vi "Compile Directional Speed 1.0 Data - Multi FPGA.vi"(7 "RIO Address":string, 8 "error in (no error)":errorcluster, 11 "Device Item Ref in":T3 format="%.0x") -> (0 "error out":errorcluster, 1 "bitfile names":string[](array[string]), 2 "Directional Speeds":T1[](array[typedef]), 3 "Device Item Ref out":T3 format="%.0x")   [LabVIEW 2015, in "Engine Simulation Toolkit System Explorer.lvlib"]
uses:
  Engine Simulation Toolkit System Explorer.lvlib
  <vilib>/NI Veristand/Custom Device API/Custom Device Item Ref.ctl
  Shared/1.0 Directional Speed Engine Data.ctl
  Shared/1.0 Directional Speed FIFO Idxs.ctl
  Digital Pattern Find Events Enum.ctl
  Custom wrapped 10 bit counter.vi
  Shared/Constants and GUIDs.vi
  <vilib>/NI Veristand/Custom Device Tools/Custom Device Utility Library/NI VeriStand - Search for Item by GUID.vi
  Shared/Properties.vi
  <vilib>/NI Veristand/Custom Device API/Get Item Property (String).vi
  <vilib>/NI Veristand/Custom Device API/Get Item Property (Dependent Node Pointer).vi
  <vilib>/NI Veristand/Custom Device Tools/Custom Device Utility Library/Custom Device Utility Library.lvlib
  Shared/Engine Simulation Toolkit Shared.lvlib
  <vilib>/NI Veristand/Custom Device API/Custom Device API.lvlib
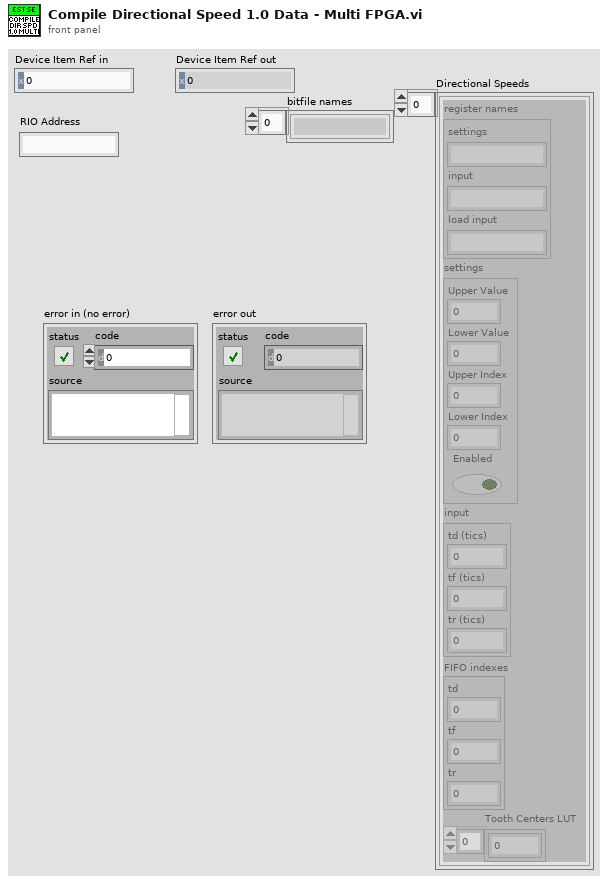
[diagram p1: front panel]
types:
  T1 = typedef "Engine Simulation Toolkit Shared.lvlib/1.0 Directional Speed Engine Data.ctl" = cluster{"register names":cluster{"settings":string, "input":string, "load input":string}, "settings":cluster{"Upper Value":u16, "Lower Value":u16, "Upper Index":fxp<+,10,10>, "Lower Index":fxp<+,10,10>, "Enabled":bool}, "input":cluster{"td (tics)":u16, "tf (tics)":u16, "tr (tics)":u16}, "FIFO indexes":T2, "Tooth Centers LUT":u16[]}
  T2 = typedef "Engine Simulation Toolkit Shared.lvlib/1.0 Directional Speed FIFO Idxs.ctl" = cluster{"td":i32, "tf":i32, "tr":i32}
  T3 = typedef "Custom Device API.lvlib/Custom Device Item Ref.ctl" = u64
  T4 = typedef "Engine Simulation Toolkit Shared.lvlib/Channel.ctl" = cluster{"Name":string, "Units":string, "Default":dbl, "Description":string, "Scalable":bool}
  T5 = typedef "Engine Simulation Toolkit System Explorer.lvlib/Digital Pattern Find Events Enum.ctl" = enum16{"Rising Edge", "Falling Edge", "Any Edge", "Center Tooth", "Center Gap"}
  T6 = typedef "Custom Device API.lvlib/Custom Device Item Info.ctl" = cluster{"Name":string, "Is Channel":bool, "GUID":string, "Is Waveform":bool}
  T7 = typedef "Engine Simulation Toolkit System Explorer.lvlib/Digital Pattern.ctl" = cluster{"Name":string, "Base":T8, "Remove":T9[], "Add":T10[], "FPGA Resource":string}
  T8 = typedef "Engine Simulation Toolkit System Explorer.lvlib/Digital Pattern Base.ctl" = cluster{"Length":dbl, "Teeth":u16, "Width":dbl, "Offset":dbl}
  T9 = typedef "Engine Simulation Toolkit System Explorer.lvlib/Digital Pattern Remove Edge.ctl" = cluster{"Tooth":u16, "Edge":bool}
  T10 = typedef "Engine Simulation Toolkit System Explorer.lvlib/Digital Pattern Add Pulse.ctl" = cluster{"Tooth":u16, "Offset":dbl, "Width":dbl}
  T11 = typedef "Engine Simulation Toolkit System Explorer.lvlib/Digital Pattern Expanded.ctl" = cluster{"X":dbl[], "Y":dbl[]}
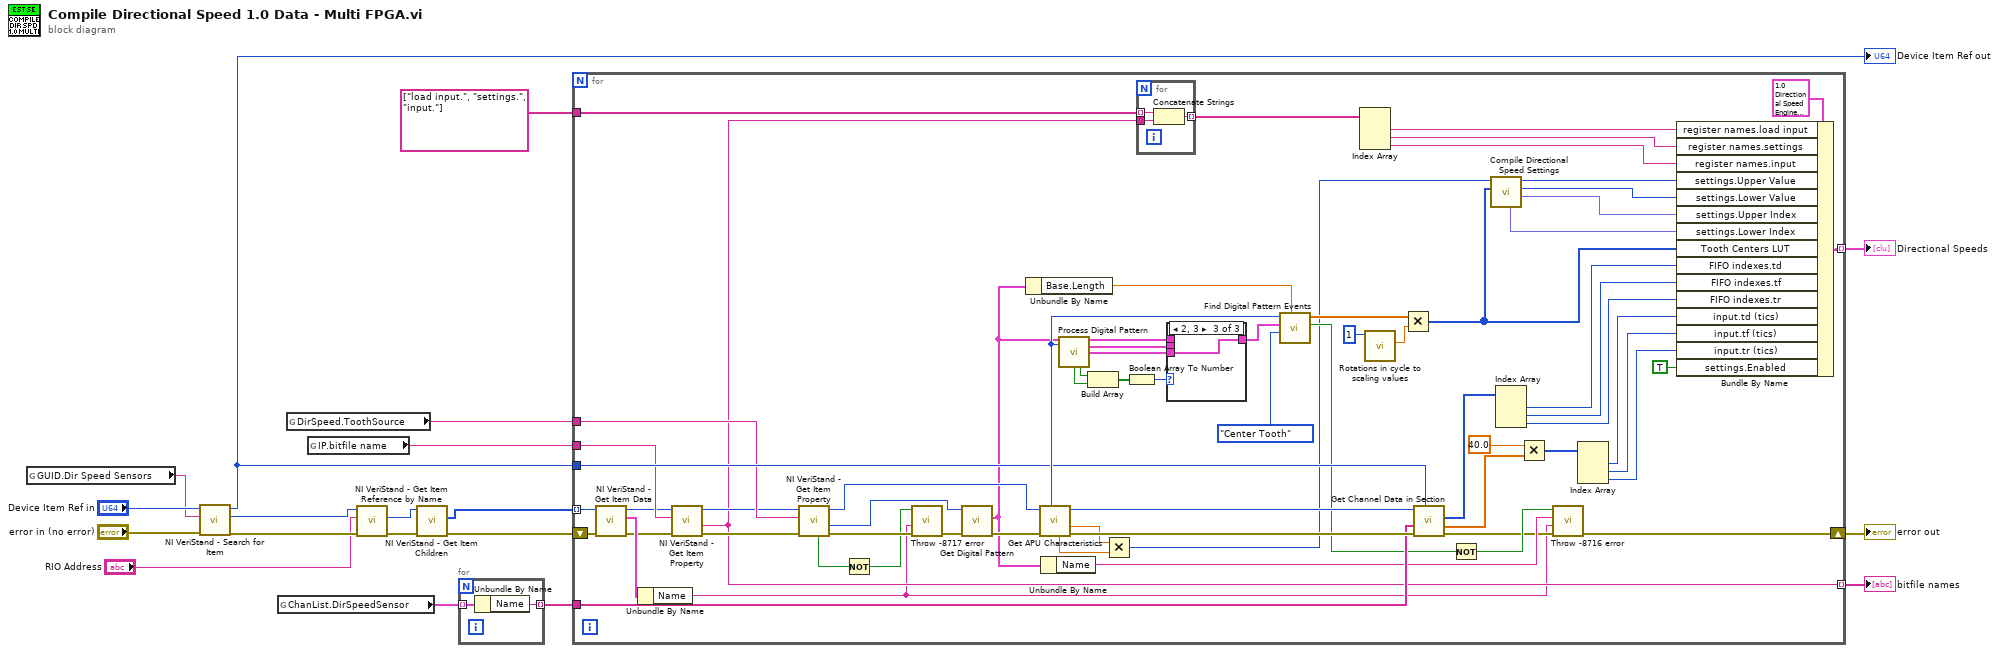
[diagram p0: block diagram]
diagram:
  n1 = global read "Constants and GUIDs.vi" "GUID.Dir Speed Sensors"() -> (w17:string)
  n2 = call-poly <vilib>:"NI VeriStand - Search for Item.vi"("error in"="error in (no error)", "Item GUID"=w17, "Section Ref in"="Device Item Ref in") -> ("error out"=w5:errorcluster, "Item Ref"=w2:T3, "Section Ref out"=w14:T3)  [unwired: 5 in, 1 out]
  "Device Item Ref out" <- w14
  n3 = global read "Constants and GUIDs.vi" "ChanList.DirSpeedSensor"() -> (w13:T4[])
  n4 = global read "Properties.vi" "DirSpeed.ToothSource"() -> (w11:string)
  n5 = global read "Properties.vi" "IP.bitfile name"() -> (w10:string)
  n6 = call <vilib>:"NI VeriStand - Get Item Reference by Name.vi"("error in (no error)"=w5, "Item Name"="RIO Address", "Parent Ref in"=w2) -> ("error out"=w7:errorcluster, "Item Ref"=w3:T3)  [unwired: 5 in, 2 out]
  n7 = call <vilib>:"NI VeriStand - Get Item Children.vi"("error in (no error)"=w7, "Item Ref in"=w3) -> ("error out"=w6:errorcluster, "Child Refs"=w4:T3[])  [unwired: 6 in, 2 out]
  n8 = for {
    tunnel: [w21] -> w12 mode=indexing
    tunnel: w13 -> [w20] mode=indexing
    n9 = Unbundle By Name(w20) -> ("Name"=w21:string)
  }
  n10 = for {
    shift-right: [w53] -> w15
    shift-left: w6 -> [w46]
    tunnel: string[] ["load input.", "settings.", "input."] -> [w59]
    tunnel: [w86] -> w8 mode=indexing
    tunnel: w14 -> [w78]
    tunnel: w4 -> [w43] mode=indexing
    tunnel: w12 -> [w77]
    tunnel: w11 -> [w64]
    tunnel: w10 -> [w55]
    tunnel: [w54] -> w9 mode=indexing
    n11 = call <vilib>:"NI VeriStand - Get Item Data.vi"("error in (no error)"=w46, "Item Ref in"=w43) -> ("error out"=w45:errorcluster, "Item Info"=w48:T6, "Item Ref out"=w44:T3)  [unwired: 6 in, 1 out]
    n12 = Unbundle By Name(w48) -> ("Name"=w39:string)
    n13 = call-poly <vilib>:"NI VeriStand - Get Item Property.vi"("error in (no error)"=w45, "Property Name"=w55, "Item Ref in"=w44) -> ("error out"=w57:errorcluster, "Value"=w54:string, "Item Ref out"=w56:T3)  [unwired: 5 in, 1 out]
    n14 = call-poly <vilib>:"NI VeriStand - Get Item Property.vi"("error in (no error)"=w57, "Property Name"=w64, "Item Ref in"=w56) -> ("error out"=w65:errorcluster, "Dependent Node Ref"=w62:T3, "Item Ref out"=w61:T3, "Found"=w41:bool)  [unwired: 5 in]
    n15 = Not(x=w41) -> (.not. x?=w40:bool)
    n16 = call "Throw -8717 error.vi"("error in (no error)"=w65, "dir speed name"=w39, "error"=w40) -> ("error out"=w42:errorcluster)  [unwired: 8 in]
    n17 = call "Get Digital Pattern.vi"("error in (no error)"=w42, "Item Ref in"=w62) -> ("error out"=w63:errorcluster, "EPT Pattern"=w50:T7)  [unwired: 7 in, 1 out]
    n18 = Unbundle By Name(w50) -> ("Base.Length"=w82:dbl)
    n19 = call "Get APU Characteristics.vi"("error in (no error)"=w63, "Item Ref in"=w61) -> ("error out"=w80:errorcluster, "angle to u16 scale factor"=w38:dbl, "Item Ref out"=w60:T3, "start angle"=w37:dbl, "rotations"=w83:u16)  [unwired: 3 in, 2 out]
    n20 = Unbundle By Name(w50) -> ("Name"=w49:string)
    n21 = call "Process Digital Pattern.vi"("EPT Pattern"=w50, "Rotations"=w83) -> ("Base"=w69:T11, 6:"Reduced"=w68:T11, 8:"Final"=w67:T11, 13:"Final"=w72:bool, 14:"Reduced"=w73:bool)  [unwired: 7 in, 2 out]
    n22 = Build Array(w73, w72) -> (w71:bool[])
    n23 = Multiply(x=w38, y=w37) -> (x*y=w36:u16)
    n24 = Boolean Array To Number(Boolean array=w71) -> (number=w70:u32)
    n25 = for {
      tunnel: w54 -> [w92]
      tunnel: w59 -> [w91] mode=indexing
      tunnel: [w90] -> w58 mode=indexing
      n26 = Concatenate Strings(w91, w92) -> (w90:string)
    }
    n27 = case shown="2, 3" w70 {
      tunnel: w69 -> [w93 _ _]
      tunnel: w68 -> [_ w94 _]
      tunnel: w67 -> [_ _ w95]
      tunnel: [w93 w94 w95] -> w66
      frame 0, Default {
      }
      frame 1 {
      }
      frame 2, 3 {
      }
    }
    n28 = call "Find Digital Pattern Events.vi"("Base.length"=w82, "Event"=Digital_Pattern_Find_Events_Enum."Center Tooth", "Pattern"=w66, "Rotations"=w83) -> ("crank angle"=w52:bool, "Locations"=w79:dbl[])  [unwired: 5 in, 1 out]
    n29 = Index Array(array=w58) -> (element #1=w88:string, element #2=w87:string, element #3=w85:string)  [unwired: 3 in]
    n30 = call "Rotations in cycle to scaling values.vi"("rotations in a cycle"=u16 1) -> ("angle to u16 scale factor"=w74:dbl)  [unwired: 8 in, 2 out]
    n31 = Multiply(x=w79, y=w74) -> (x*y=w31:u16[])
    n32 = call "Get Channel Data in Section.vi"("Custom device ref"=w78, "error in (no error)"=w80, "Channels"=w77, "Item Ref in"=w60) -> ("error out"=w47:errorcluster, "default values"=w75:dbl[], "FIFO indexes"=w76:i32[])  [unwired: 3 in, 2 out]
    n33 = Not(x=w52) -> (.not. x?=w51:bool)
    n34 = call "Compile Directional Speed Settings.vi"("Tooth centers"=w31, "APU start position"=w36) -> ("upper index"=w33:fxp<+,10,10>, "lower value"=w34:u16, "upper value"=w35:u16, "lower index"=w32:fxp<+,10,10>)  [unwired: 6 in]
    n35 = Index Array(array=w76) -> (element #1=w30:i32, element #2=w29:i32, element #3=w28:i32)  [unwired: 3 in]
    n36 = Multiply(x=40.0 ("rotations in a cycle"), y=w75) -> (x*y=w27:u16[])
    n37 = call "Throw -8716 error.vi"("error in (no error)"=w47, "dir speed name"=w39, "tooth source name"=w49, "error"=w51) -> ("error out"=w53:errorcluster)  [unwired: 7 in]
    n38 = Index Array(array=w27) -> (element #1=w25:u16, element #2=w24:u16, element #3=w23:u16)  [unwired: 3 in]
    n39 = Bundle By Name(cluster=T1 {"register names"={"settings"="", "input"="", "load input"=""}, "settings"={"Upper Value"=0, "Lower Value"=0, "Upper Index"=0.0, "Lower Index"=0.0, "Enabled"=FALSE}, "input"={"td (tics)"=0, "tf (tics)"=0, "tr (tics)"=0}, "FIFO indexes"={"td"=0, "tf"=0, "tr"=0}, "Tooth Centers LUT"=[]} ("1.0.0 Directional Speed"), "register names.load input"=w88, "register names.settings"=w87, "register names.input"=w85, "settings.Upper Value"=w35, "settings.Lower Value"=w34, "settings.Upper Index"=w33, "settings.Lower Index"=w32, "Tooth Centers LUT"=w31, "FIFO indexes.td"=w30, "FIFO indexes.tf"=w29, "FIFO indexes.tr"=w28, "input.td (tics)"=w25, "input.tf (tics)"=w24, "input.tr (tics)"=w23, "settings.Enabled"=TRUE) -> (w86:T1)
  }
  "error out" <- w15
  "Directional Speeds" <- w8
  "bitfile names" <- w9
